vi "Read_Data_Json.vi"(8 "error in (no error)":errorcluster caption="entrée d'erreur (pas d'erreur)", 11 "Firebase AssembledProducts en entrée":refnum<class "Firebase AssembledProducts.lvclass">) -> (0 "error out":errorcluster caption="sortie d'erreur", 2 "Data":string, 3 "Firebase AssembledProducts en sortie":refnum<class "Firebase AssembledProducts.lvclass">)   [LabVIEW 2020, in "Library Instrument & Equipement.lvlib" / "Library FireBase.lvlib" / "Firebase AssembledProducts.lvclass"]
uses:
  Firebase AssembledProducts.lvclass
  Firebase AssembledProducts.lvclass/Firebase AssembledProducts.ctl
  JSON API/Variant JSON/Variant to JSON.vi
  JSON API/JSON Value/Get Item by name array.vi
  JSON API/JSON Value/JSON Value.lvclass
  JSON API/Get Polymorphic/JSON GetSet.lvlib
  JSON API/Variant JSON/Variant JSON.lvlib
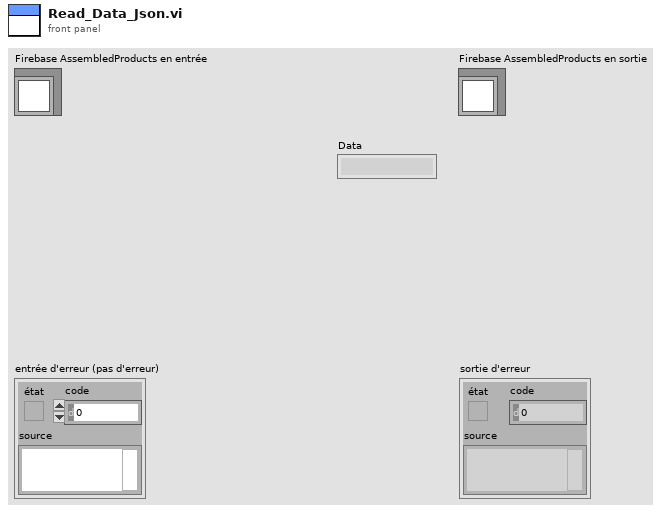
[diagram p1: front panel]
types:
  T1 = cluster{"name":string, "fields":cluster{"Result":cluster{"booleanValue":bool}, "CreationDate":cluster{"timestampValue":string}, "Batch":cluster{"stringValue":string}, "SerialNumber":cluster{"stringValue":string}, "EndOfProduction":cluster{"timestampValue":string}, "FW_Version":cluster{"mapValue":cluster{"fields":cluster{"Bootloader":cluster{"mapValue":cluster{"fields":cluster{"File_Name":cluster{"stringValue":string}, "Version":cluster{"mapValue":cluster{"fields":cluster{"Major":cluster{"stringValue":string}, "Minor":cluster{"stringValue":string}}}}, "Checksum":cluster{"stringValue":string}}}}, "SoftDevice":cluster{"mapValue":cluster{"fields":cluster{"File_Name":cluster{"stringValue":string}, "Version":cluster{"mapValue":cluster{"fields":cluster{"Major":cluster{"stringValue":string}, "Minor":cluster{"stringValue":string}}}}, "Checksum":cluster{"stringValue":string}}}}, "DFU":cluster{"mapValue":cluster{"fields":cluster{"File_Name":cluster{"stringValue":string}, "Version":cluster{"mapValue":cluster{"fields":cluster{"Major":cluster{"stringValue":string}, "Minor":cluster{"stringValue":string}}}}, "Checksum":cluster{"stringValue":string}}}}}}}, "PartNumber":cluster{"stringValue":string}, "OrderNumber":cluster{"stringValue":string}, "Operator":cluster{"stringValue":string}, "AssembledProductName":cluster{"stringValue":string}}}[]
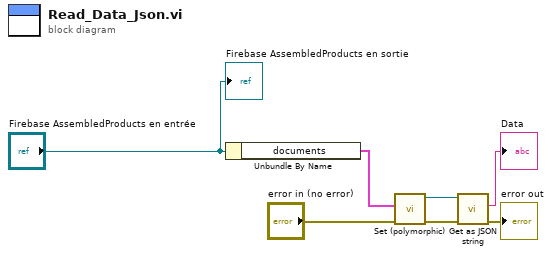
[diagram p0: block diagram]
diagram:
  n1 = Unbundle By Name("Firebase AssembledProducts en entrée") -> ("documents"=w5:T1)
  n2 = call-poly "Set (polymorphic).vi"("error in (no error)"="error in (no error)", "Variant"=w5) -> ("error out"=w6:errorcluster, "JSON Value out"=w7:refnum<class "JSON Value.lvclass">)  [unwired: 8 in]
  n3 = call "Get as JSON string.vi"("error in (no error)"=w6, "JSON Value in"=w7) -> ("error out"=→"error out":errorcluster, "<JSON>"=→"Data":string)  [unwired: 8 in]
  "Firebase AssembledProducts en sortie" <- "Firebase AssembledProducts en entrée"
